vi "Read rotIPA.vi"(8 "error in (no error)":errorcluster, 11 "CurrentRotatorPositions in":refnum<class "CurrentRotatorPositions.lvclass">) -> (0 "error out":errorcluster, 2 "rotIPA":dbl[unit] min=-6.283185307179586 max=6.283185307179586, 3 "CurrentRotatorPositions out":refnum<class "CurrentRotatorPositions.lvclass">)   [LabVIEW 2014, in "TCSDataDefinitions.lvlib" / "TCSPublicStatus.lvlib" / "PointingPositions.lvlib" / "CurrentRotatorPositions.lvclass"]
uses:
  CurrentRotatorPositions.lvclass
  CurrentRotatorPositions.lvclass/CurrentRotatorPositions.ctl
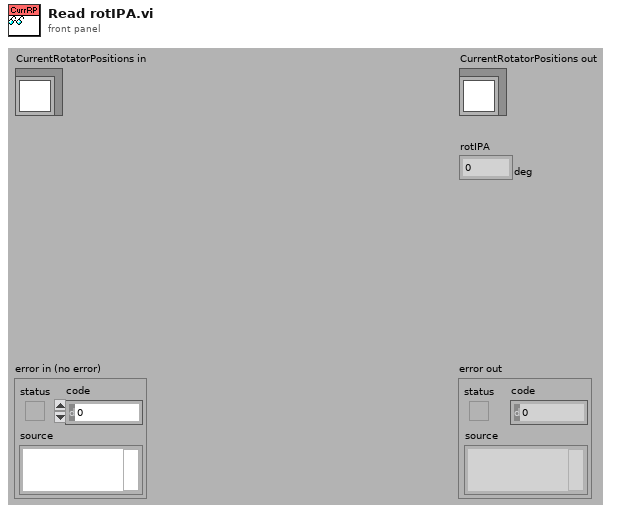
[diagram p1: front panel]
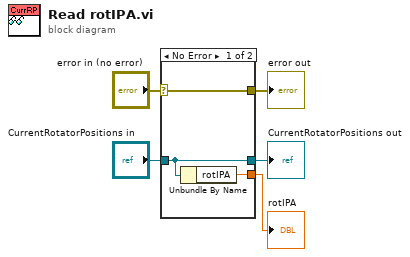
[diagram p0: block diagram]
diagram:
  n1 = case shown="No Error" "error in (no error)" {
    selector: "error in (no error)" -> [w8 w9]
    tunnel: [w8 w9] -> w4
    tunnel: [w7 w10] -> w2
    tunnel: "CurrentRotatorPositions in" -> [w7 w10]
    tunnel: [w6 _] -> w1
    frame No Error {
      n2 = Unbundle By Name(w7) -> ("rotIPA"=w6:dbl[unit])
    }
    frame Error {
    }
  }
  "error out" <- w4
  "CurrentRotatorPositions out" <- w2
  "rotIPA" <- w1
